vi "Destruct.vi"(8 "error in (no error)":errorcluster, 11 "muExpr in":refnum<class "Tag Expr.lvclass">) -> (0 "error out":errorcluster)   [LabVIEW 2020, in "Tag Expr.lvclass"]
doc: "Destruct the muExpr instance. This will release the muParser handle and variable pointers."
uses:
  Tag Expr.lvclass
  Tag Expr.lvclass/Tag Expr.ctl
  <vilib>/LAVA/muParser/mupExpr/mupExpr.lvclass
panel:
  # "Destruct the muExpr instance. This will release the muParser handle and variable pointers."
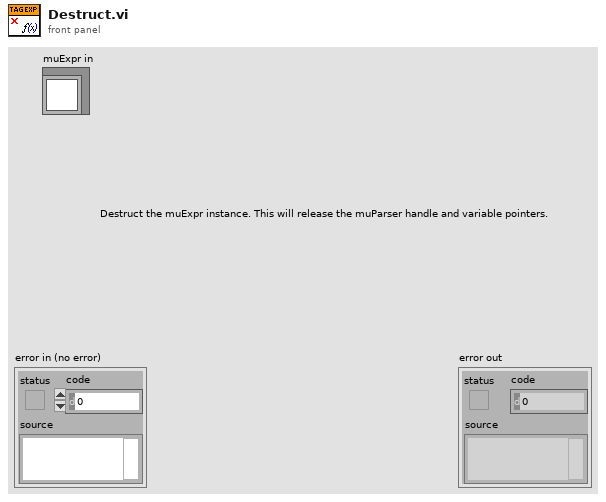
[diagram p1: front panel]
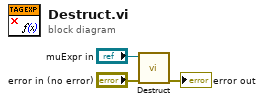
[diagram p0: block diagram]
diagram:
  n1 = call-parent "Destruct.vi"("error in (no error)"="error in (no error)", "muExpr in"="muExpr in") -> ("error out"=→"error out":errorcluster)  [unwired: 9 in]
